vi "Acceptable Measurement.vi"(1 "Main Dose Calibration Cluster":T1={"Dose Response"={"grand_mean"=0.0372961188, "slope"=0.0115712882}, "Dose Correction"={"Sex"=1, "a0"=7.719669421, "a1"=-2.746550736, "a2"=-0.186490355, "a3"=0.041922063, "a4"=-0.849147359, "a5"=0.14330063, "a6"=0.019930219, "A_n"=40.0, "H_n"=10.95, "Dose Correction"=TRUE}, "Dose Reporting"={"Reporting is"=TRUE, "sd_threshold [AU]"=0.06, "sd_model [Gy]"=0.66, "dosimetric_threshold [Gy]"=2.0, "Add intrasession errors is"=TRUE, "Prior Radiation?"=TRUE}} {"Dose Reporting"."dosimetric_threshold [Gy]" format="%#_9g"; "Dose Reporting"."sd_model [Gy]" format="%#_9g"; "Dose Reporting"."sd_threshold [AU]" format="%#_9g"; "Dose Correction"."H_n" format="%#_9g"; "Dose Correction"."A_n" format="%#_9g"; "Dose Correction"."a6" format="%#.9g"; "Dose Correction"."a5" format="%#.9g"; "Dose Correction"."a4" format="%#.9g"; "Dose Correction"."a3" format="%#.9g"; "Dose Correction"."a2" format="%#.9g"; "Dose Correction"."a1" format="%#.9g"; "Dose Correction"."a0" format="%#.9g"; "Dose Correction"."Sex" items=["Male"=1, "Female"=0]; "Dose Response"."slope" format="%#_9g"; "Dose Response"."grand_mean" format="%#_9g"}, 2 "Set RIS Estimates [AU]":dbl[](array[numeric])=[0.02, 0.03, 0.04, 0.04, 0.03] format="%#_9g") -> (0 "Acceptable Measurement":bool)   [LabVIEW 2016]
uses:
  Dose Calculation Control.ctl
  <vilib>/Analysis/NI_AALBase.lvlib
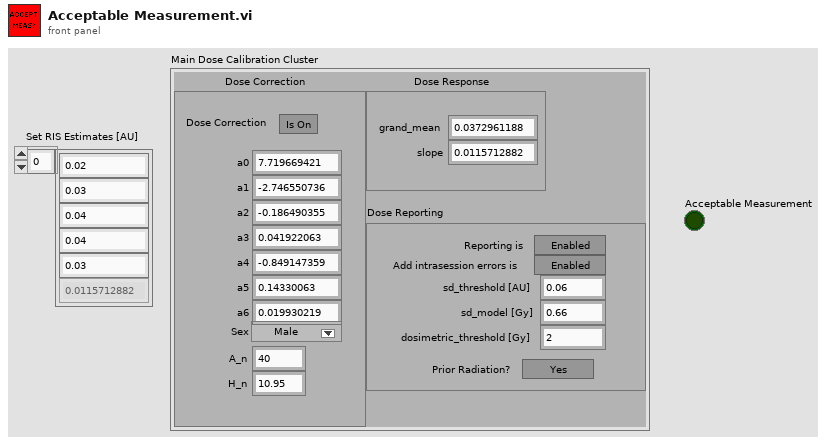
[diagram p1: front panel]
types:
  T1 = typedef "Dose Calculation Control.ctl" = cluster{"Dose Response":cluster{"grand_mean":dbl, "slope":dbl}, "Dose Correction":cluster{"Sex":u16, "a0":dbl, "a1":dbl, "a2":dbl, "a3":dbl, "a4":dbl, "a5":dbl, "a6":dbl, "A_n":dbl, "H_n":dbl, "Dose Correction":bool}, "Dose Reporting":cluster{"Reporting is":bool, "sd_threshold [AU]":dbl, "sd_model [Gy]":dbl, "dosimetric_threshold [Gy]":dbl, "Add intrasession errors is":bool, "Prior Radiation?":bool}}
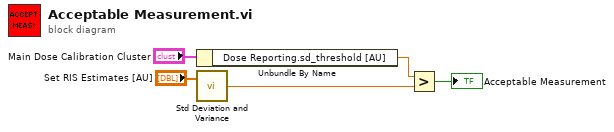
[diagram p0: block diagram]
diagram:
  n1 = Unbundle By Name("Main Dose Calibration Cluster") -> ("Dose Reporting.sd_threshold [AU]"=w3:dbl)
  n2 = call <vilib>:"Std Deviation and Variance.vi"("X"="Set RIS Estimates [AU]") -> ("standard deviation"=w2:dbl)  [unwired: 1 in, 2 out]
  n3 = Greater?(x=w3, y=w2) -> (0:→"Acceptable Measurement":bool)
